vi "SaveLot_New.vi"(8 "error in (no error)":errorcluster, 11 "LotData in":refnum<class "LotData.lvclass">) -> (0 "error out":errorcluster, 2 "Message":string, 3 "LotData out":refnum<class "LotData.lvclass">)   [LabVIEW 2012, in "LotData.lvclass"]
uses:
  LotData.lvclass
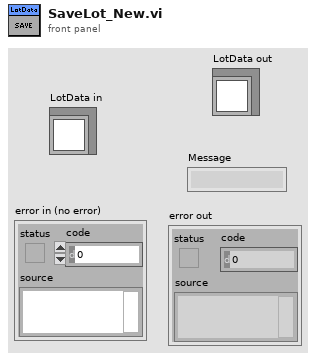
[diagram p1: front panel]
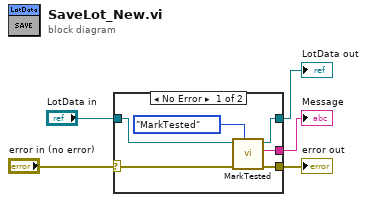
[diagram p0: block diagram]
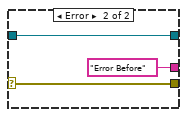
[diagram p2: hidden frame]
diagram:
  n1 = case shown="No Error" "error in (no error)" {
    selector: "error in (no error)" -> [w6 w14]
    tunnel: [w11 w14] -> w4
    tunnel: [w10 w13] -> w2
    tunnel: "LotData in" -> [w7 w13]
    tunnel: [w9 "Error Before" ("Message")] -> w1
    frame No Error {
      n2 = call-dynamic "MarkTested.vi"("Enum"=enum16{"MarkTested", "MarkNotTested"}."MarkTested", "error in (no error)"=w6, "LotData in"=w7) -> ("error out"=w11:errorcluster, "Message"=w9:string, "LotData out"=w10:refnum<class "LotData.lvclass">)  [unwired: 6 in]
    }
    frame Error {
    }
  }
  "error out" <- w4
  "LotData out" <- w2
  "Message" <- w1
